vi "File Dialog__jki_lib_file -- VI Tester.vi"(0 "start path":path, 1 "prompt":string, 5 "selection mode (existing file)":T1(ring), 7 "pattern label":string, 9 "default name":string, 11 "pattern":string, 13 "button label":string) -> (4 "path":path, 6 "Paths":path[](array[path]), 10 "exists":bool, 15 "cancelled":bool)   [LabVIEW 2011]
doc: "This VI behaves the same way as the built-in LabVIEW file dialog except that this one remembers the last path that was used when it was called.\n\nYou can use this dialog box to select existing files or directories or to select a location and name for a new file or directory.\n\nprompt is the message that appears below the list of files and directories in the dialog box. prompt defaults to an empty string if unwired.\n start path is the path of the directory whose contents LabVIEW initially displays in the dialog box. If start path is valid, but does not refer to an existing directory, LabVIEW strips names from the end of the path until the path is a valid directory path or an empty path. If start path is invalid or unwired, the last directory viewed in a file dialog initially appears in the dialog box.\n\nselect mode indicates the types of files or directories you can specify using the dialog box. select mode defaults to 2 if you do not wire it.\n\n0 Select only an existing file. You might use this value if you want the user to select the name of a file to open; the program can then open the file using the Open File function. \n1 Select only a file that does not exist. You might use this value if you want the user to select the name of a file to create; the program can then create the file using the New File function.\n2 Select either an existing or a non-existent file. You might use this value if you want the user to select the name of a file to create or append data to. This is the default if you leave select mode unwired.\n3 Select only an existing directory. You might use this value if you want the user to select the name of a directory that contains data files. The program can then access those files with the directory path.\n4 Select only a non-existent directory. You might use this value if you want the user to select the name of a directory that the program subsequently creates using the New Directory function.\n5 Select either an existing or a non-existent directory. You might use this value if you want the user to select the name of a directory in which to store data files. The program can create the directory if it does not exist. \n6 Select an existing file in an LLB.\n7 Select a new file in an LLB.\n8 Select an existing or new file in an LLB.\ndefault name is the name you want to appear as the initial file or directory name in the dialog box. This parameter defaults to the empty string if unwired.\n pattern optionally restricts the files displayed in the dialog box to those whose name matches pattern. pattern does not restrict the directories displayed in the dialog box. The pattern matching performed here is similar to the one used in matching wildcards in Windows and UNIX file names and not like the regular expression matching performed by the Match Pattern function. If you specify characters other than the question mark character ( ? ) or the asterisk character ( * ), the File Dialog function displays only files or directories that contain those characters. You can use the question mark character ( ? ) to match any single character. You can use the asterisk character ( * ) to match any sequence of one or more characters. \n\nFor example, a pattern input of *.vi;test*.llb returns matches for any file with a .vi extension and any file whose filename begins with test and has an .llb extension.\n To match multiple patterns, use a semicolon ( ; ) to separate the patterns. White space, such as blanks, tabs, and carriage returns, are taken literally. Avoid using white spaces unless they are part of the extension pattern. For example, if you use \"*.html;*.doc\", File Dialog displays all files that end with .html and .doc. If you use \"*.html; *.doc\", File Dialog displays only files that end with .html. \n\nTo use more than one pattern, wire a string constant or control into file pattern\n datalog type can be wired to any data type. If wired, it restricts the files displayed in the dialog box to datalog files containing records of the specified data type.\n path is the full path to the file or directory selected using this dialog box. If you select Cancel, this function sets path to Not A Path.\n exists is TRUE if path specifies an existing file or directory.\n\ncancelled is TRUE if you close the dialog box by selecting Cancel or if an error occurs during the execution of the dialog box."
uses:
  <userlib>/_OpenG.lib/file/file.llb/Valid Path - Traditional__ogtk.vi
  <vilib>/Utility/config.llb/Read Key (Path).vi
  <vilib>/Utility/config.llb/Write Key (Path).vi
  <vilib>/Utility/config.llb/NI_LVConfig.lvlib
panel:
  out "error out":errorcluster
  # "Copyright © 2006 James Kring, Inc. All rights reserved.\nMichael Aivaliotis michael.aivaliotis@jameskring.com\nalternate email: michael@aivaliotis.com\n\nThis library is provided \"AS IS\" , WITHOUT WARRANTIES OR \nCONDITIONS OF ANY KIND, either express or implied.\n\nJames Kring, Inc. -- http://www.jameskring.com"
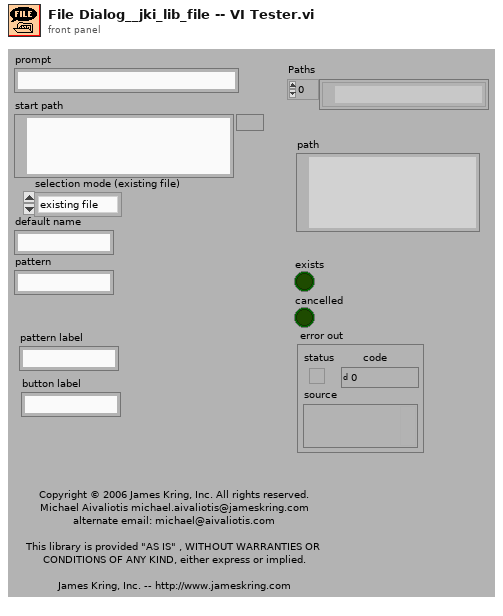
[diagram p1: front panel]
types:
  T1 = enum32{"existing file", "new file", "new or existing file", "existing dir", "new dir", "new or existing dir", "existing file (use LLBs)", "new file (use LLBs)", "new or existing file (use LLBs)", "new or existing file or directory (use LLBs)", "existing dir (use LLBs)", "new dir (use LLBs)", "new or existing dir (use LLBs)", "existing file or dir", "new file or dir", "new or existing file or dir", "existing file or dir (use LLBs)", "new file or dir (use LLBs)", "multi-select", "multi-select (use LLBs)"}
  T2 = typedef "NI_LVConfig.lvlib/Config Data RefNum.ctl" = refnum<k1>
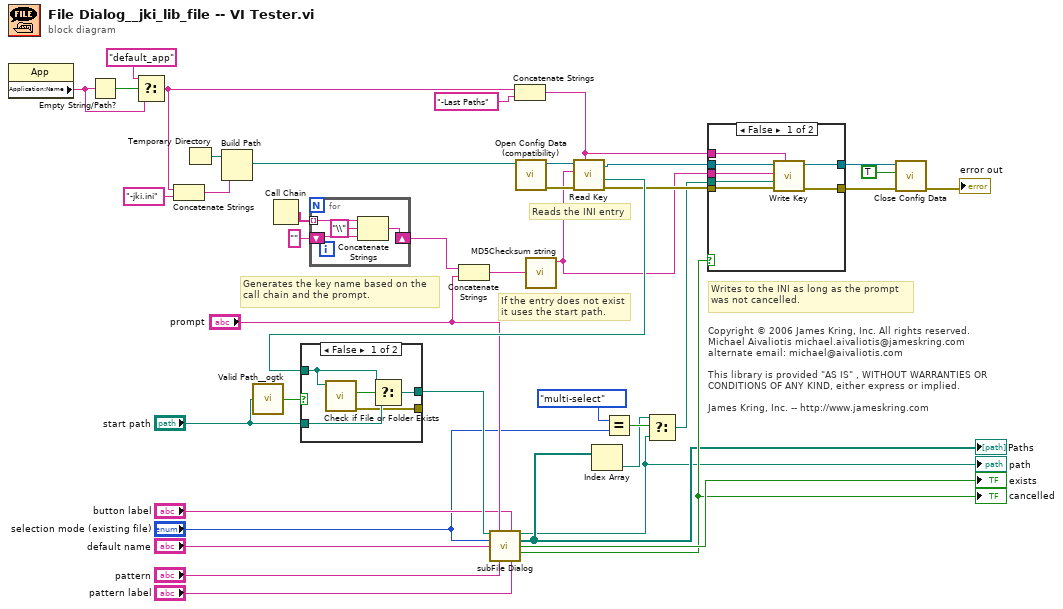
[diagram p0: block diagram]
diagram:
  # "Copyright © 2006 James Kring, Inc. All rights reserved.\nMichael Aivaliotis michael.aivaliotis@jameskring.com\nalternate email: michael@aivaliotis.com\n\nThis library is provided \"AS IS\" , WITHOUT WARRANTIES OR \nCONDITIONS OF ANY KIND, either express or implied.\n\nJames Kring, Inc. -- http://www.jameskring.com"
  # "Writes to the INI as long as the prompt\nwas not cancelled."
  # "If the entry does not exist it uses the start path."
  # "Generates the key name based on the\ncall chain and the prompt."
  # "Reads the INI entry"
  n1 = property class="App"() -> ("Application:Name"=w10:string)  [unwired: 2 in, 2 out]
  n2 = Empty String/Path?(string/path=w10) -> (empty?=w7:bool)
  n3 = Select(t="default_app", s=w7, f=w10) -> (s? t:f=w2:string)
  n4 = Concatenate Strings(w2, "-jki.ini" ("name or relative path")) -> (w1:string)
  n5 = Temporary Directory() -> (w5:path)
  n6 = Build Path(base path=w5, name or relative path=w1) -> (appended path=w4:path)
  n7 = call-poly <userlib>:"Valid Path__ogtk.vi"("path"="start path") -> ("valid"=w11:bool)
  n8 = Call Chain() -> (call chain=w41:string[])
  n9 = for {
    tunnel: w41 -> [w43] mode=indexing
    shift-right: [w45] -> w39
    shift-left: "" -> [w42]
    n10 = Concatenate Strings(w43, "\\" ("Input Element"), w42) -> (w45:string)
  }
  n11 = Concatenate Strings(w39, "prompt") -> (w29:string)
  n12 = Concatenate Strings(w2, "-Last Paths" ("section (empty)")) -> (w6:string)
  n13 = call <vilib>:"Open Config Data (compatibility).vi"("configuration file path"=w4) -> ("error out"=w36:errorcluster, "refnum"=w38:T2)  [unwired: 8 in, 1 out]
  n14 = call <vilib>:"MD5Checksum string.vi"("Message String"=w29) -> ("MD5 message-digest"=w28:string)  [unwired: 10 in]
  n15 = call-poly <vilib>:"Read Key.vi"("section"=w6, "error in (no error)"=w36, "key"=w28, "refnum"=w38) -> ("error out"=w35:errorcluster, "value"=w37:path, "refnum out"=w34:T2)  [unwired: 4 in, 1 out]
  n16 = case shown="False" w11 {
    tunnel: w37 -> [w49 _]
    tunnel: [w48 w51] -> w27
    tunnel: "start path" -> [w47 w51]
    tunnel: [w46 _] -> _
    frame False {
      n17 = call <vilib>:"Check if File or Folder Exists.vi"("path"=w49) -> ("error out"=w46:errorcluster, "file or folder exists?"=w50:bool)  [unwired: 8 in, 1 out]
      n18 = Select(t=w49, s=w50, f=w47) -> (s? t:f=w48:path)
    }
    frame True {
    }
  }
  n19 = call <vilib>:"subFile Dialog.vi"("start path"=w27, "prompt"="prompt", "button label"="button label", "selection mode"="selection mode (existing file)", "default name"="default name", "pattern (all files)"="pattern", "pattern label"="pattern label") -> ("selected path"=w13:path, "selected paths"=w17:path[], "exists"=→"exists":bool, "cancelled"=w21:bool)  [unwired: 4 in, 1 out]
  "path" <- w13
  "cancelled" <- w21
  "Paths" <- w17
  n20 = Index Array(array=w17) -> (element=w15:path)  [unwired: 1 in]
  n21 = Equal?(x=T1."multi-select", y="selection mode (existing file)") -> (x = y?=w16:bool)
  n22 = Select(t=w15, s=w16, f=w13) -> (s? t:f=w14:path)
  n23 = case shown="False" w21 {
    tunnel: w35 -> [w58 w59]
    tunnel: w34 -> [w57 w60]
    tunnel: [w56 w59] -> w33
    tunnel: [w55 w60] -> w31
    tunnel: w6 -> [w54 _]
    tunnel: w28 -> [w53 _]
    tunnel: w14 -> [w52 _]
    frame False {
      n24 = call-poly <vilib>:"Write Key.vi"("section"=w54, "error in (no error)"=w58, "value"=w52, "key"=w53, "refnum"=w57) -> ("error out"=w56:errorcluster, "refnum out"=w55:T2)  [unwired: 4 in, 1 out]
    }
    frame True {
    }
  }
  n25 = call <vilib>:"Close Config Data.vi"("error in (no error)"=w33, "write file if changed (T)"=TRUE ("write configuration file? (F)"), "refnum"=w31) -> ("error out"=→"error out":errorcluster)  [unwired: 7 in, 1 out]
